vi "ErrorHandling.Append.vi"(7 "new error code (0: unchanged)":i32=5000, 8 "error in":errorcluster, 10 "append text":string) -> (0 "error out":errorcluster)   [LabVIEW 2013]
doc: "Creates an error in the error wire.\nIf an error is present in <B>error in</B>, it will be passed on without any further action.\n\nOnly actually creates the error if <B>create</B>=True (default).\nIn the text of the error the source VI and call trace is added, as well as the time.\n\nA message that you could attach to the <B>explanation</B> input could be the following lines:\n Invalid config file format.\n File: C:\\myapp\\savetheworld.ini"
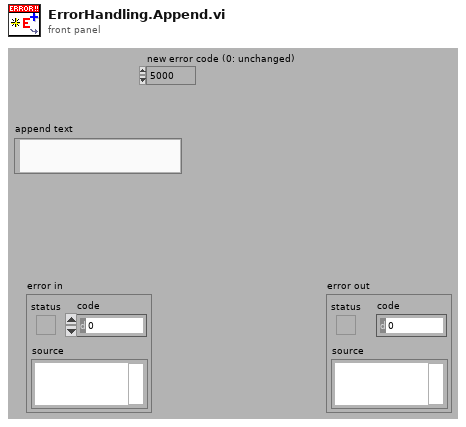
[diagram p1: front panel]
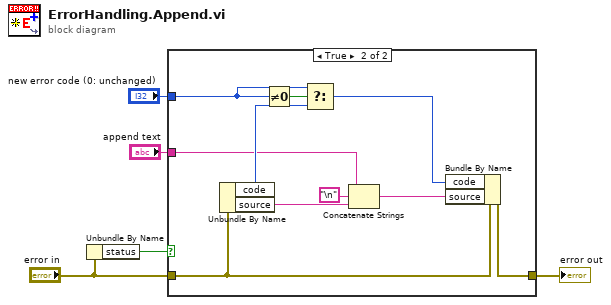
[diagram p0: block diagram]
diagram:
  n1 = Unbundle By Name("error in") -> ("status"=w2:bool)
  n2 = case shown="True" w2 {
    tunnel: [w6 w16] -> w5
    tunnel: "error in" -> [w6 w12]
    tunnel: "append text" -> [_ w7]
    tunnel: "new error code (0: unchanged)" -> [_ w9]
    frame False {
    }
    frame True {
      n3 = Unbundle By Name(w12) -> ("code"=w10:i32, "source"=w15:string)
      n4 = Not Equal To 0?(x=w9) -> (x != 0?=w11:bool)
      n5 = Select(t=w9, s=w11, f=w10) -> (s? t:f=w8:i32)
      n6 = Concatenate Strings(w7, "\n", w15) -> (w13:string)
      n7 = Bundle By Name(cluster=w12, "code"=w8, "source"=w13) -> (w16:errorcluster)
    }
  }
  "error out" <- w5
